vi "纳清余氯_所有参数读取.vi"(8 "error in (no error)":errorcluster caption="错误输入（无错误）", 11 "MB session in":refnum<class "MB_Master.lvclass">) -> (0 "error out":errorcluster caption="错误输出", 2 "输出值":T1, 3 "MB session out":refnum<class "MB_Master.lvclass">)   [LabVIEW 2022 SP3, in "斯坦道多参数.lvlib"]
uses:
  <vilib>/Plasmionique/MB Master/MB_Master/MB_Master.lvclass
  <vilib>/Plasmionique/MB Master/MB Master.lvlib
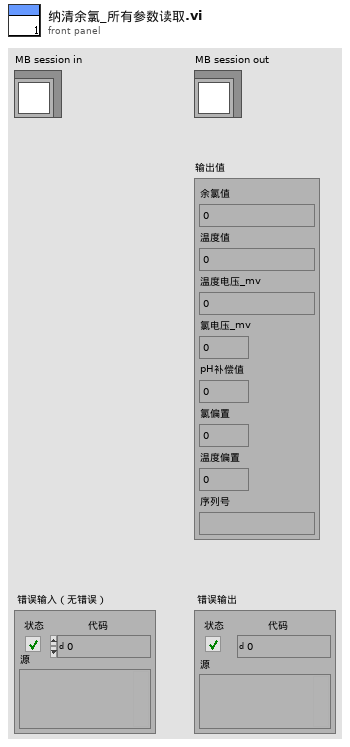
[diagram p1: front panel]
types:
  T1 = cluster{"余氯值":sgl, "温度值":sgl, "温度电压_mv":sgl, "氯电压_mv":dbl, "pH补偿值":dbl, "氯偏置":dbl, "温度偏置":dbl, "序列号":string}
  T2 = cluster{"pH":u32, "DO":u32, "Cond":u32, "Turb":u32, "叶绿素a":u32, "藻密度":u32, "ORP":u32, "COD":u32, "氯化物":u32, "氨氮":u32, "水中油":u32, "悬浮物":u32, "余氯":u32}
  T3 = cluster{"mode":dbl, "数值":sgl, "数值":sgl, "数值":sgl, "数值":sgl, "数值":sgl, "数值":sgl, "类型":string}
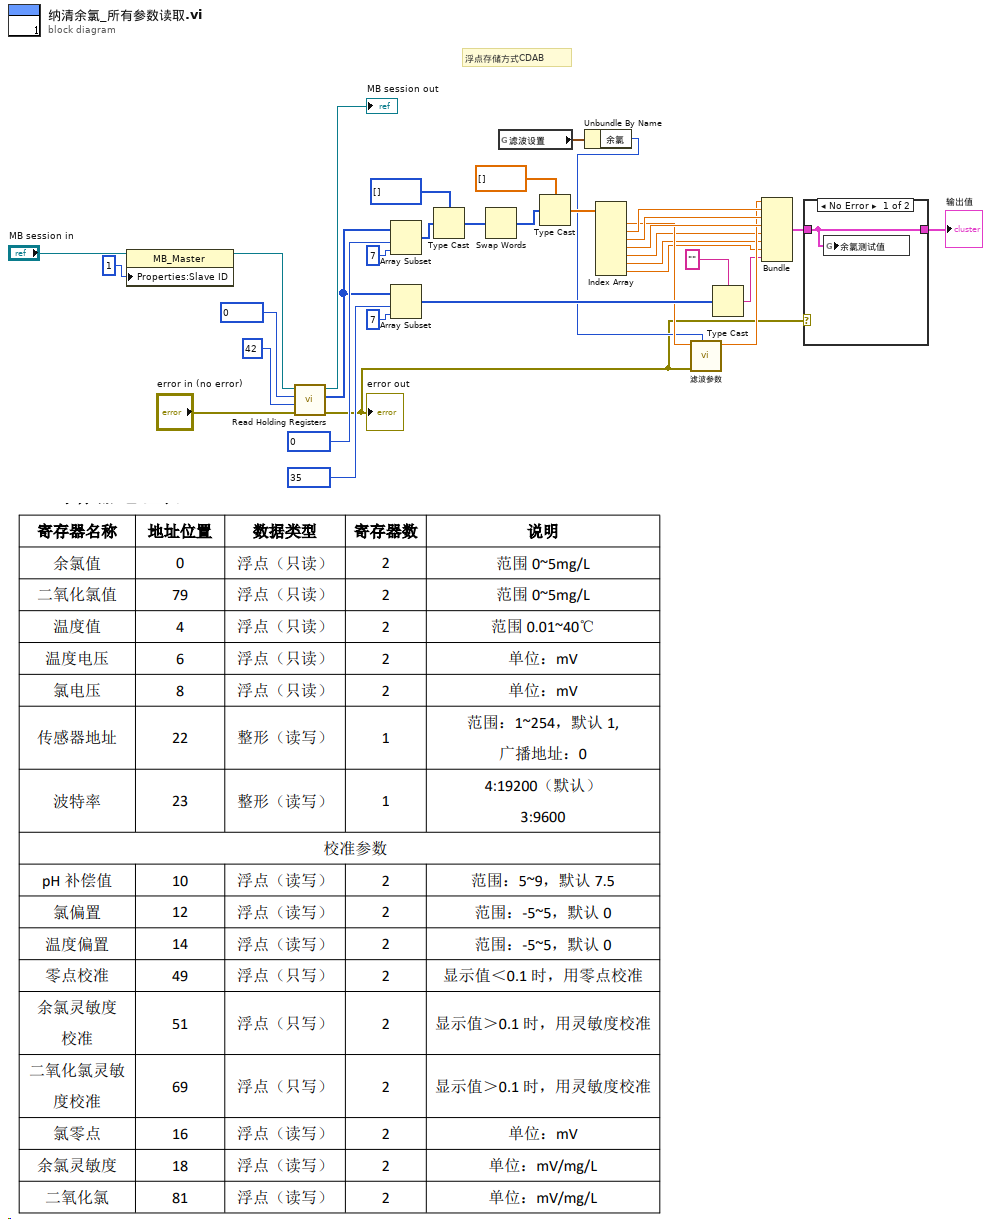
[diagram p0: block diagram]
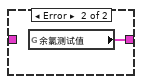
[diagram p2: hidden frame]
diagram:
  # "浮点存储方式CDAB"
  n1 = property class="MB_Master"(reference="MB session in", "Properties:Slave ID"=u8 1 ("Slave ID")) -> (reference out=w25:refnum<class "MB_Master.lvclass">)  [unwired: 1 in, 1 out]
  n2 = call <vilib>:"Read Holding Registers.vi"("error in (no error)"="error in (no error)", "quantity"=u16 42, "starting address"=u16 0, "MB session in"=w25) -> ("error out"=w7:errorcluster, "Registers"=w5:u16[], "MB session out"=→"MB session out":refnum<class "MB_Master.lvclass">)  [unwired: 5 in]
  "error out" <- w7
  n3 = Array Subset(array=w5, index=u16 0 ("starting address"), length=7 ("长度")) -> (w29:u16[])
  n4 = Array Subset(array=w5, index=u16 35 ("starting address"), length=7 ("长度")) -> (w20:u16[])
  n5 = Type Cast(type=u32[] [] ("数组 2"), x=w29) -> (*(type *) &x=w18:u32[])
  n6 = Swap Words(1:w18) -> (0:w6:u32[])
  n7 = global read "断电保存变量.vi" "滤波设置"() -> (w10:T2)
  n8 = Type Cast(type=sgl[] [] ("数组 2"), x=w6) -> (*(type *) &x=w28:sgl[])
  n9 = Unbundle By Name(w10) -> ("余氯"=w9:u32)
  n10 = Index Array(array=w28) -> (element #1=w12:sgl, element #2=w23:sgl, element #3=w15:sgl, element #4=w14:sgl, element #5=w4:sgl, element #6=w3:sgl, element #7=w2:sgl)  [unwired: 7 in]
  n11 = call "滤波参数.vi"("滤波次数"=w9, "error in (no error)"=w7, "x"=w12) -> ("mode"=w11:dbl)  [unwired: 7 in, 1 out]
  n12 = Type Cast(type="" ("类型"), x=w20) -> (*(type *) &x=w1:string)
  n13 = Bundle("mode"=w11, "数值"=w23, "数值"=w15, "数值"=w14, "数值"=w4, "数值"=w3, "数值"=w2, "类型"=w1) -> (w13:T3)  [unwired: 1 in]
  n14 = case shown="No Error" w7 {
    tunnel: w13 -> [w35 _]
    tunnel: [w35 w36] -> w8
    frame No Error {
      n15 = global write "纳清过程全局变量.vi" "余氯测试值"(w35) -> ()
    }
    frame Error {
      n16 = global read "纳清过程全局变量.vi" "余氯测试值"() -> (w36:T1)
    }
  }
  "输出值" <- w8
